vi "get offset.vi"(8 "error in (no error)":errorcluster, 11 "Thorcam in":refnum<class "Thorcam.lvclass">) -> (0 "error out":errorcluster, 3 "Thorcam out":refnum<class "Thorcam.lvclass">)   [LabVIEW 2012, in "Thorcam.lvclass"]
uses:
  Thorcam.lvclass
  Thorcam.lvclass/Thorcam.ctl
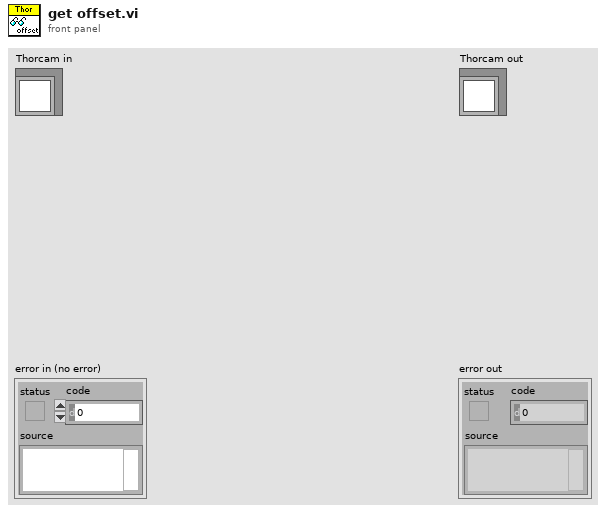
[diagram p1: front panel]
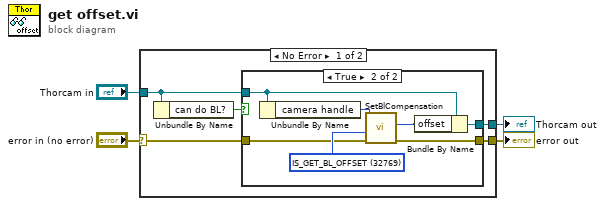
[diagram p0: block diagram]
diagram:
  n1 = case shown="No Error" "error in (no error)" {
    selector: "error in (no error)" -> [w8 w20]
    tunnel: [w7 w20] -> w3
    tunnel: [w5 w19] -> w1
    tunnel: "Thorcam in" -> [w6 w19]
    frame No Error {
      n2 = Unbundle By Name(w6) -> ("can do BL?"=w9:bool)
      n3 = case shown="True" w9 {
        tunnel: w6 -> [w11 w13]
        tunnel: w8 -> [w10 w16]
        tunnel: [w10 w15] -> w7
        tunnel: [w11 w12] -> w5
        frame False {
        }
        frame True {
          w18 = 32769 items=["IS_BL_COMPENSATION_DISABLE"=0, "IS_BL_COMPENSATION_ENABLE"=1, "IS_GET_BL_COMPENSATION"=32768, "IS_GET_BL_OFFSET"=32769, "IS_GET_BL_DEFAULT_MODE"=32770, "IS_GET_BL_DEFAULT_OFFSET"=32771, "IS_GET_BL_SUPPORTED_MODE"=32772, "IS_IGNORE_PARAMETER"=-1] ("Mode")
          n4 = Unbundle By Name(w13) -> ("camera handle"=w17:u32)
          n5 = call <instrlib>:"SetBlCompensation.vi"("error in"=w16, "Mode"=w18, "Camera Handle In"=w17) -> ("error out"=w15:errorcluster, "Value"=w14:i32)  [unwired: 6 in, 1 out]
          n6 = Bundle By Name(cluster=w13, "offset"=w14) -> (w12:refnum<class "Thorcam.lvclass">)
        }
      }
    }
    frame Error {
    }
  }
  "error out" <- w3
  "Thorcam out" <- w1
